vi "查询启动项.vi"(8 "error in (no error)":errorcluster caption="错误输入（无错误）") -> (0 "error out":errorcluster caption="错误输出", 3 "包含启动项":bool)   [LabVIEW 2016, in "Alarm interface.lvlib" / "wxpusher.lvlib"]
uses:
  wxpusher.lvlib
  <vilib>/registry/registry.llb/Registry RtKey.ctl
  <vilib>/registry/registry.llb/Registry SAM.ctl
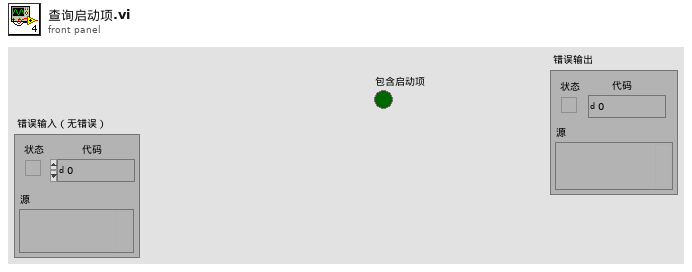
[diagram p1: front panel]
types:
  T1 = typedef "Registry SAM.ctl" = enum32{"KEY_QUERY_VALUE", "KEY_SET_VALUE", "KEY_CREATE_SUB_KEY", "KEY_ENUMERATE_SUB_KEYS", "KEY_NOTIFY", "KEY_CREATE_LINK", "KEY_READ", "KEY_WRITE", "KEY_ALL_ACCESS", "KEY_READ | KEY_WRITE"}
  T2 = typedef "Registry RtKey.ctl" = enum32{"HKEY_CLASSES_ROOT", "HKEY_CURRENT_USER", "HKEY_LOCAL_MACHINE", "HKEY_USERS", "HKEY_PERFORMANCE_DATA", "HKEY_CURRENT_CONFIG", "HKEY_DYN_DATA"}
  T3 = typedef "Registry refnum.ctl" = refnum<k1>
  T4 = cluster{"numValues":i32, "maxValueNameLen":i32, "maxValueDataLen":i32}
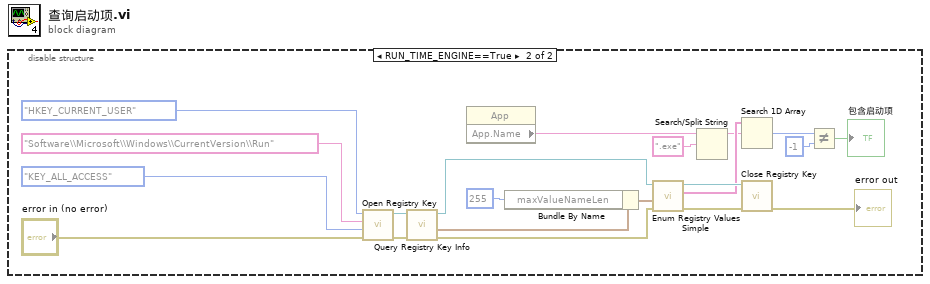
[diagram p0: block diagram]
diagram:
  n1 = disable-structure shown="RUN_TIME_ENGINE==True" {
    frame condition #0 (active) {
    }
    frame condition #1 {
      n2 = call <vilib>:"Open Registry Key.vi"("error in (no error)"="error in (no error)", "security access mask (KEY_READ | KEY_WRITE)"=Registry_SAM."KEY_ALL_ACCESS", "subkey"="Software\\Microsoft\\Windows\\CurrentVersion\\Run", "root key (HKEY_LOCAL_MACHINE)"=Registry_RtKey."HKEY_CURRENT_USER") -> ("error out"=w18:errorcluster, "refnum out"=w19:T3)  [unwired: 6 in]
      n3 = call <vilib>:"Query Registry Key Info.vi"("error in (no error)"=w18, "refnum"=w19) -> ("error out"=w15:errorcluster, "value info"=w16:T4, "refnum out"=w17:T3)  [unwired: 5 in, 2 out]
      n4 = property class="App"() -> ("App.Name"=w4:string)  [unwired: 2 in, 2 out]
      n5 = Bundle By Name(cluster=w16, "maxValueNameLen"=255) -> (w2:T4)
      n6 = call <vilib>:"Enum Registry Values Simple.vi"("error in (no error)"=w15, "value info"=w2, "refnum"=w17) -> ("error out"=w13:errorcluster, "values"=w12:string[], "refnum out"=w14:T3)  [unwired: 3 in, 3 out]
      n7 = Search/Split String(string=w4, search string/char (-)=".exe" ("搜索字符串/字符(-)")) -> (substring before match=w3:string)  [unwired: 1 in, 2 out]
      n8 = Search 1D Array(1D array=w12, element=w3) -> (index of element=w11:i32)  [unwired: 1 in]
      n9 = call <vilib>:"Close Registry Key.vi"("error in (no error)"=w13, "refnum"=w14) -> ("error out"=→"error out":errorcluster)  [unwired: 5 in]
      n10 = Not Equal?(x=w11, y=-1) -> (x != y?=→"包含启动项":bool)
    }
  }
